vi "Start.vi"(8 "error in":errorcluster, 10 "WFM in":waveform(dbl)[](array[waveform]), 11 "DAQmx in":refnum<class "DAQmx.lvclass">) -> (0 "error out":errorcluster, 3 "DAQmx out":refnum<class "DAQmx.lvclass">)   [LabVIEW 2019, in "DAQmx.lvclass"]
uses:
  DAQmx.lvclass
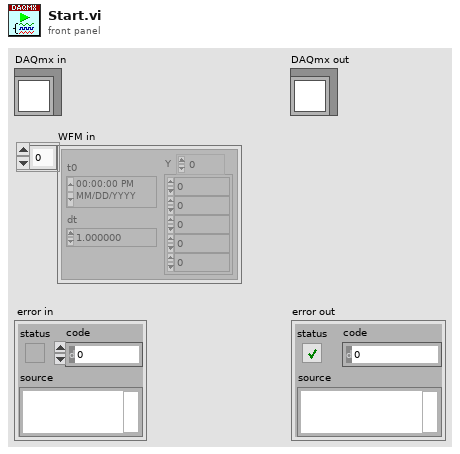
[diagram p1: front panel]
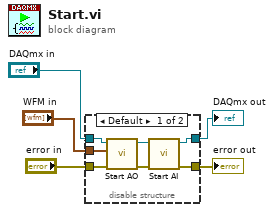
[diagram p0: block diagram]
diagram:
  n1 = disable-structure shown="Default" {
    disable-tunnel: "DAQmx in" -> [w7 w14]
    disable-tunnel: "error in" -> [w6 w13]
    disable-tunnel: [w10 w14] -> w3
    disable-tunnel: [w9 w13] -> w2
    disable-tunnel: "WFM in" -> [w8 _]
    frame condition #0 (active) {
      n2 = call "Start AO.vi"("error in (no error)"=w6, "AO []"=w8, "DAQmx in"=w7) -> ("error out"=w12:errorcluster, "DAQmx out"=w11:refnum<class "DAQmx.lvclass">)  [unwired: 7 in]
      n3 = call "Start AI.vi"("error in (no error)"=w12, "DAQmx in"=w11) -> ("error out"=w9:errorcluster, "DAQmx out"=w10:refnum<class "DAQmx.lvclass">)  [unwired: 6 in]
    }
    frame condition #1 {
    }
  }
  "error out" <- w2
  "DAQmx out" <- w3
